vi "MDAQ_IndexProgress.vi"(10 "Input Cluster":T1 {"CV"."Temperature Array" scale=0.0..100.0}) -> (2 "output cluster":T1 {"CV"."Temperature Array" scale=0.0..100.0}, 5 "Selected Amplitude":dbl)   [LabVIEW 2021]
uses:
  GUI_Def.ctl
  Mode_Enum.ctl
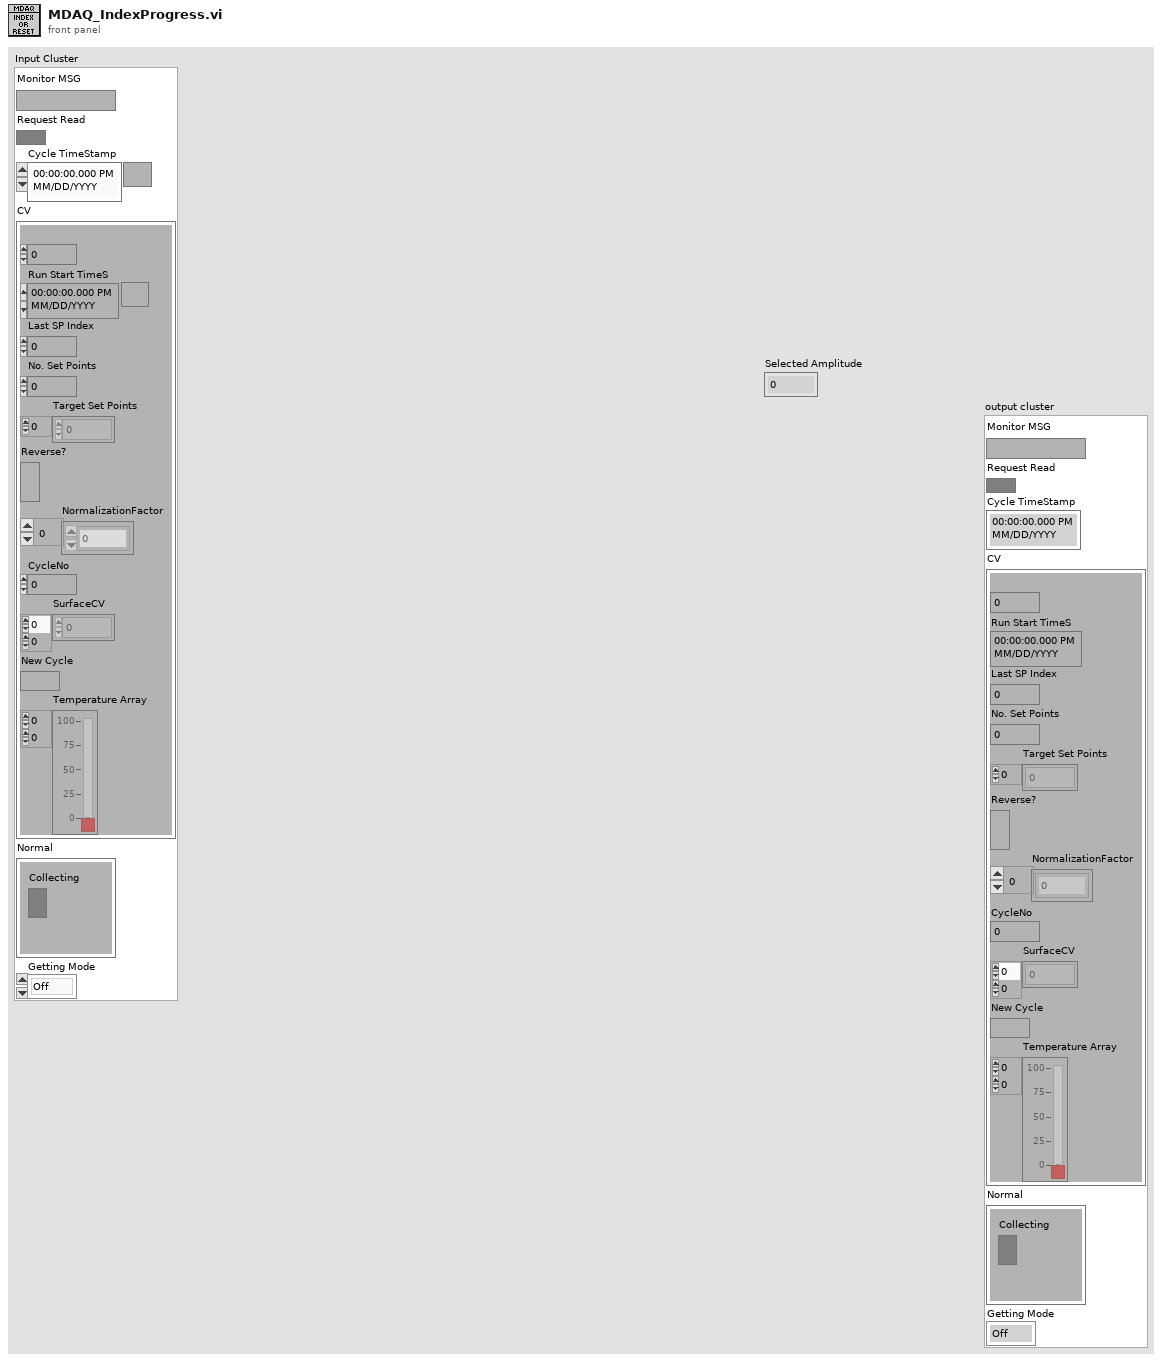
[diagram p1: front panel]
types:
  T1 = typedef "GUI_Def.ctl" = cluster{"Monitor MSG":string, "Request Read":bool, "Cycle TimeStamp":timestamp, "CV":cluster{"Set Point Index":u32, "Run Start TimeS":timestamp, "Last SP Index":u32, "No. Set Points":u32, "Target Set Points":i32[], "Reverse?":bool, "NormalizationFactor":i32[], "CycleNo":i32, "SurfaceCV":dbl[][], "New Cycle":bool, "Temperature Array":dbl[][]}, "Normal":cluster{"Collecting":bool}, "Getting Mode":T2}
  T2 = typedef "Mode_Enum.ctl" = enum16{"Off", "Normal", "CV+Temp", "CV"}
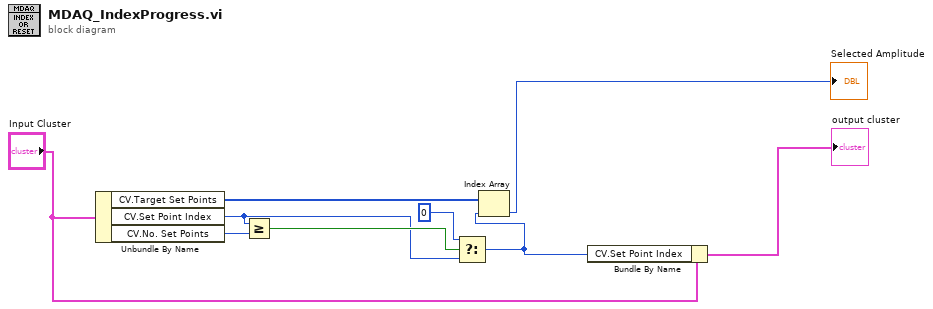
[diagram p0: block diagram]
diagram:
  n1 = Unbundle By Name("Input Cluster") -> ("CV.Target Set Points"=w9:i32[], "CV.Set Point Index"=w3:u32, "CV.No. Set Points"=w8:u32)
  n2 = Greater Or Equal?(x=w3, y=w8) -> (x >= y?=w7:bool)
  n3 = Select(t=u32 0, s=w7, f=w3) -> (s? t:f=w2:u32)
  n4 = Index Array(array=w9, index=w2) -> (element=→"Selected Amplitude":i32)
  n5 = Bundle By Name(cluster="Input Cluster", "CV.Set Point Index"=w2) -> (→"output cluster":T1)
